vi "Obtain Broadcast Events for Registration.vi"(8 "error in (no error)":errorcluster) -> (0 "error out":errorcluster, 2 "Already running?":bool, 3 "FlexiFlowInterface Broadcast Events":T1)   [LabVIEW 2024, in "FlexiFlowInterface.lvlib"]
doc: "Return the broadcast event refnums so the module's caller can register for the module's broadcast events.\n_____\nBased on Delacor QMH Project Template 3.1.0.34."
uses:
  FlexiFlowInterface.lvlib
  Broadcast Events--cluster.ctl
  Did Init Argument--cluster.ctl
  Status Updated Argument--cluster.ctl
  Error Reported Argument--cluster.ctl
  Stop Argument--cluster.ctl
  Get Module Execution Status Argument--cluster.ctl
  Broadcast Device States Argument--cluster.ctl
  Modbus Flexi-Flow State--cluster.ctl
  <vilib>/Plasmionique/MB Master/MB_Master_TCP/MB_Master_TCP.lvclass
  Device Type--enum.ctl
  Modbus Flexi-Flow Controls--cluster.ctl
  Modbus Flexi-Flow API/Control Mode--enum.ctl
  Modbus Flexi-Flow API/Control Function Values--enum.ctl
  Modbus Flexi-Flow Measure State--cluster.ctl
  Broadcast State (Data Map) Argument--cluster.ctl
  Modbus Flexi-Flow API/Bronkhorst Flexi-Flow ModbusTCP API.lvlib
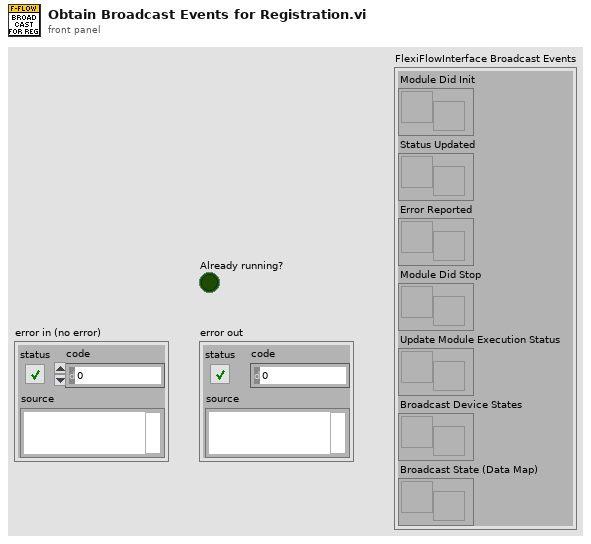
[diagram p1: front panel]
types:
  T1 = typedef "FlexiFlowInterface.lvlib/Broadcast Events--cluster.ctl" = cluster{"Module Did Init":refnum<user-event>, "Status Updated":refnum<user-event>, "Error Reported":refnum<user-event>, "Module Did Stop":refnum<user-event>, "Update Module Execution Status":refnum<user-event>, "Broadcast Device States":refnum<user-event>, "Broadcast State (Data Map)":refnum<user-event>}
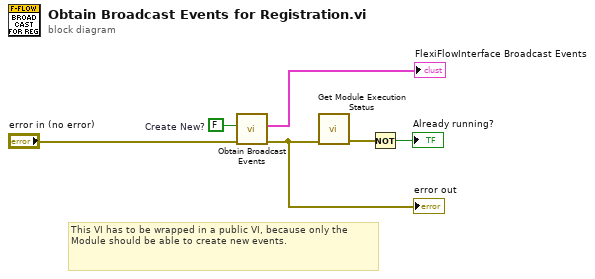
[diagram p0: block diagram]
diagram:
  w5 = FALSE  # Create New?
  # "This VI has to be wrapped in a public VI, because only the Module should be able to create new events."
  n1 = call "Obtain Broadcast Events.vi"("error in (no error)"="error in (no error)", "Create New?"=w5) -> ("error out"=w3:errorcluster, "FlexiFlowInterface Broadcast Events"=→"FlexiFlowInterface Broadcast Events":T1)  [unwired: 8 in]
  "error out" <- w3
  n2 = call "Get Module Execution Status.vi"("error in (no error)"=w3) -> ("error out"=w2:errorcluster)  [unwired: 10 in]
  n3 = Not(x=w2) -> (.not. x?=→"Already running?":bool)
